vi "ConvertFalconDriveEncoders.vi"(0 "Shifter State":T1(ring), 9 "Position (Raw Sensor Units)":i32, 11 "Velocity (Raw Sensor Units per 100 ms)":i32, 12 "Shift Time Threshold (ms)":u32, 13 "Latched Shift Time (ms)":u32) -> (8 "Transitioning":bool, 10 "Position (in)":dbl, 15 "Velocity (ft/s)":dbl)   [LabVIEW 2020]
doc: "This VI converts the raw Falcon 500/Talon FX encoder postion and velocity data into units of inches and feet per second, respectively. Handles low and high gear ratios."
uses:
  4f28cd8e-abc6-4562-a814-960cbb5a26e1.vi
  GlobalDrivebase.vi
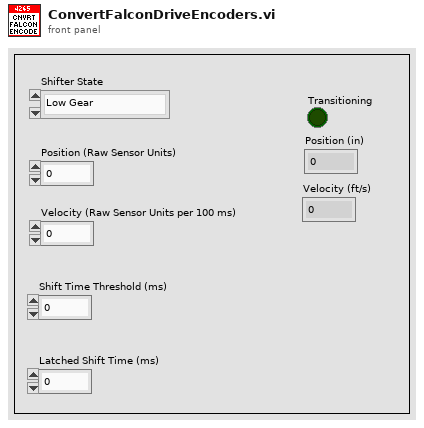
[diagram p1: front panel]
types:
  T1 = enum16{"Low Gear", "High Gear", "Transiting", "Unknown", "Force Low Gear"}
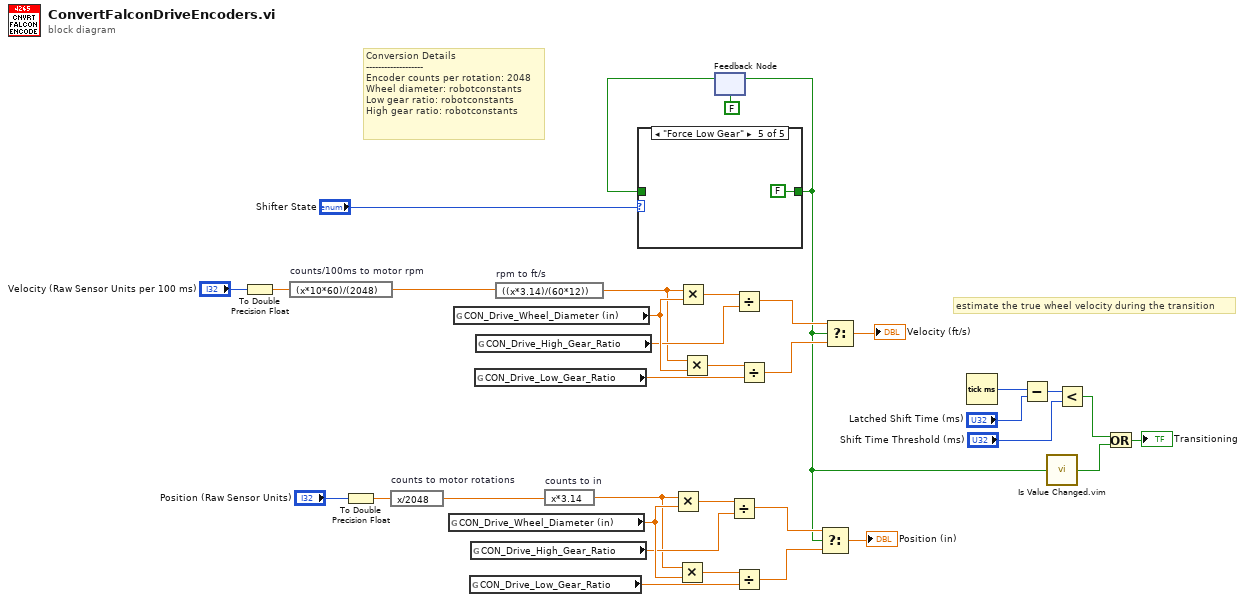
[diagram p0: block diagram]
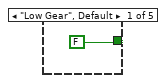
[diagram p2: hidden frame]
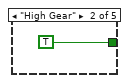
[diagram p3: hidden frame]
diagram:
  # "estimate the true wheel velocity during the transition"
  # "Conversion Details\n-------------------\nEncoder counts per rotation: 2048\nWheel diameter: robotconstants\nLow gear ratio: robotconstants\nHigh gear ratio: robotconstants"
  n1 = To Double Precision Float(number="Velocity (Raw Sensor Units per 100 ms)") -> (double precision float=w32:dbl)
  n2 = expression code="(x*10*60)/(2048)" "counts/100ms to motor rpm"(w32) -> (w30:dbl)
  n3 = To Double Precision Float(number="Position (Raw Sensor Units)") -> (double precision float=w18:dbl)
  n4 = expression code="x/2048" "counts to motor rotations"(w18) -> (w15:dbl)
  n5 = global read "GlobalDrivebase.vi" "CON_Drive_Wheel_Diameter (in)"() -> (w10:dbl)
  n6 = global read "GlobalDrivebase.vi" "CON_Drive_Wheel_Diameter (in)"() -> (w21:dbl)
  n7 = global read "GlobalDrivebase.vi" "CON_Drive_Low_Gear_Ratio"() -> (w8:dbl)
  n8 = global read "GlobalDrivebase.vi" "CON_Drive_High_Gear_Ratio"() -> (w9:dbl)
  n9 = global read "GlobalDrivebase.vi" "CON_Drive_Low_Gear_Ratio"() -> (w19:dbl)
  n10 = global read "GlobalDrivebase.vi" "CON_Drive_High_Gear_Ratio"() -> (w20:dbl)
  n11 = expression code="((x*3.14)/(60*12))" "rpm to ft/s"(w30) -> (w16:dbl)
  n12 = expression code="x*3.14" "counts to in"(w15) -> (w7:dbl)
  n13 = Multiply(x=w7, y=w10) -> (x*y=w14:dbl)
  n14 = Multiply(x=w7, y=w10) -> (x*y=w12:dbl)
  n15 = Multiply(x=w16, y=w21) -> (x*y=w25:dbl)
  n16 = Multiply(x=w16, y=w21) -> (x*y=w23:dbl)
  n17 = feedback #1(FALSE) -> (w34:bool)
  n18 = case shown="\"Force Low Gear\"" "Shifter State" {
    tunnel: [FALSE TRUE w38 w39 FALSE] -> w5
    tunnel: w34 -> [_ _ w38 w39 _]
    frame "Low Gear", Default {
    }
    frame "High Gear" {
    }
    frame "Transiting" {
    }
    frame "Unknown" {
    }
    frame "Force Low Gear" {
    }
  }
  n19 = feedback-in #1(w5) -> ()
  n20 = Divide(x=w14, y=w9) -> (x/y=w13:dbl)
  n21 = Divide(x=w25, y=w20) -> (x/y=w24:dbl)
  n22 = Divide(x=w12, y=w8) -> (x/y=w11:dbl)
  n23 = Divide(x=w23, y=w19) -> (x/y=w22:dbl)
  n24 = Select(t=w13, s=w5, f=w11) -> (s? t:f=→"Position (in)":dbl)
  n25 = Select(t=w24, s=w5, f=w22) -> (s? t:f=→"Velocity (ft/s)":dbl)
  n26 = Tick Count (ms)() -> (millisecond timer value=w29:u32)
  n27 = Subtract(x=w29, y="Latched Shift Time (ms)") -> (x-y=w28:u32)
  n28 = call "Is Value Changed.vim"("value"=w5) -> ("changed or first call?"=w1:bool)
  n29 = Less?(x=w28, y="Shift Time Threshold (ms)") -> (x < y?=w3:bool)
  n30 = Or(x=w3, y=w1) -> (x .or. y?=→"Transitioning":bool)
